vi "Settings.vi"(11 "Error In":errorcluster) -> (3 "Male/Female":T1=enum."Male", 4 "Subject Out":string, 6 "Condtion Out":string, 8 "Random Trials":bool, 10 "Visual Feedback Out":bool, 13 "Baloon Delay (ms) Out":u32, 15 "Error Out":errorcluster)   [LabVIEW 2018, in "CollectionSupport.lvlib"]
uses:
  CollectionSupport.lvlib
  Controls/Male_Female.ctl
panel:
  in  "Balloon Delay (ms)":u32
  in  "Subject":string
  in  "Condtion":string
  in  "Random Trials":bool
  in  "Visual Feedback":bool
  in  "OK Button":bool
  in  "Sex":T1=enum."Male"
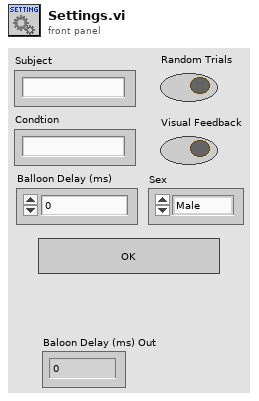
[diagram p1: front panel]
types:
  T1 = typedef "CollectionSupport.lvlib/Male_Female.ctl" = enum16{"Female", "Male"}
  T2 = enum8{"Enabled", "Disabled", "Disabled and Grayed Out"}
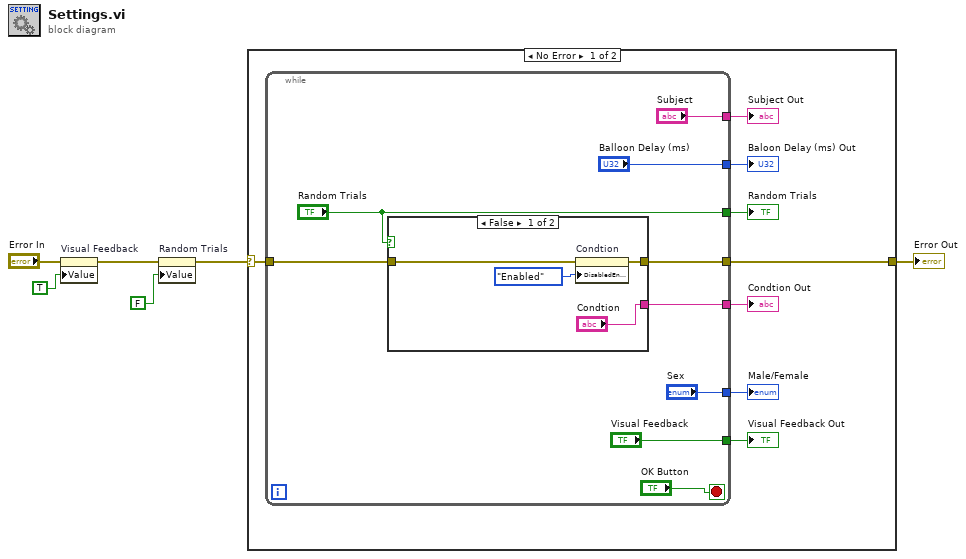
[diagram p0: block diagram]
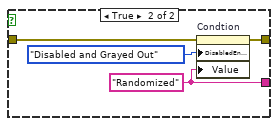
[diagram p2: hidden frame]
diagram:
  n1 = property on="Visual Feedback" class="Bool (strict)"(error in="Error In", "Value"=TRUE ("Visual Feedback")) -> (error out=w3:errorcluster)  [unwired: 1 in, 1 out]
  n2 = property on="Random Trials" class="Bool (strict)"(error in=w3, "Value"=FALSE ("Random Trials")) -> (error out=w2:errorcluster)  [unwired: 1 in, 1 out]
  n3 = case shown="No Error" w2 {
    selector: w2 -> [w14 w32]
    tunnel: [w13 w32] -> w6
    frame No Error {
      n4 = while {
        tunnel: w14 -> [w16]
        tunnel: [w15] -> w13
        tunnel: ["Visual Feedback"] -> w12
        tunnel: ["Sex"] -> w11
        tunnel: ["Balloon Delay (ms)"] -> w10
        tunnel: [w17] -> w9
        tunnel: ["Random Trials"] -> w8
        tunnel: ["Subject"] -> w7
        stop <- "OK Button" stop-if-true
        n5 = case shown="False" "Random Trials" {
          tunnel: ["Condtion" w28] -> w17
          tunnel: w16 -> [w26 w30]
          tunnel: [w25 w29] -> w15
          frame False {
            n6 = property on="Condtion" class="Str"(error in=w26, "DisabledEnum"=T2."Enabled" ("Disabled")) -> (error out=w25:errorcluster)  [unwired: 1 in, 1 out]
          }
          frame True {
            w28 = "Randomized" ("Condtion")
            n7 = property on="Condtion" class="Str"(error in=w30, "DisabledEnum"=T2."Disabled and Grayed Out" ("Disabled"), "Value"=w28) -> (error out=w29:errorcluster)  [unwired: 1 in, 1 out]
          }
        }
      }
      "Subject Out" <- w7
      "Random Trials" <- w8
      "Condtion Out" <- w9
      "Baloon Delay (ms) Out" <- w10
      "Male/Female" <- w11
      "Visual Feedback Out" <- w12
    }
    frame Error {
    }
  }
  "Error Out" <- w6
